vi "Set Topmost.vi"(8 "error in (no error)":errorcluster, 10 "Topmost":bool, 11 "GVIWebProcessorApp in":refnum<class "GVIWebProcessorApp.lvclass">) -> (0 "error out":errorcluster, 3 "GVIWebProcessorApp out":refnum<class "GVIWebProcessorApp.lvclass">)   [LabVIEW 2020, in "PicoG-Processor.lvlib" / "GVIWebProcessorApp.lvclass"]
uses:
  GVIWebProcessorApp.lvclass
  <vilib>/Utility/error.llb/Error Cluster From Error Code.vi
  <vilib>/ErrorRing/Error Ring.xnode
  PicoG-Processor.lvlib
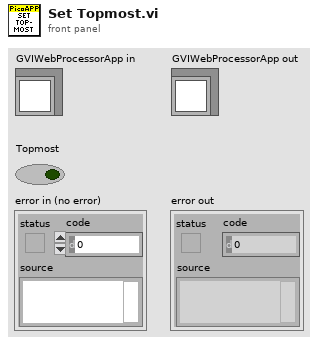
[diagram p1: front panel]
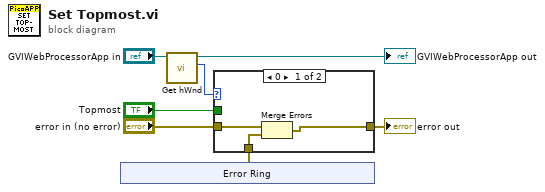
[diagram p0: block diagram]
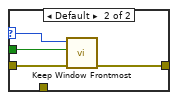
[diagram p2: hidden frame]
diagram:
  n1 = xnode "Error Ring"() -> ("error out"=w3:errorcluster)
  n2 = call "Get hWnd.vi"("GVIWebProcessorApp in"="GVIWebProcessorApp in") -> ("hWnd"=w5:i32, "GVIWebProcessorApp out"=→"GVIWebProcessorApp out":refnum<class "GVIWebProcessorApp.lvclass">)  [unwired: 8 in, 1 out]
  n3 = case shown="0" w5 {
    selector: w5 -> [_ w13]
    tunnel: "error in (no error)" -> [w10 w14]
    tunnel: [w8 w12] -> w4
    tunnel: w3 -> [w9 _]
    tunnel: "Topmost" -> [_ w11]
    frame 0 {
      n4 = Merge Errors(w10, w9) -> (w8:errorcluster)
    }
    frame Default {
      n5 = call "Keep Window Frontmost.vi"("error in (no error)"=w14, "Topmost?"=w11, "hWnd"=w13) -> ("error out"=w12:errorcluster)  [unwired: 8 in]
    }
  }
  "error out" <- w4
